vi "Add Subscriber.vi"(8 "error in (no error)":errorcluster, 10 "New FIFO Instance Config":T1, 11 "CIF_DAQ_DVR_Multi in":refnum<class "CIF_NIChn_DAQ.lvclass">) -> (0 "error out":errorcluster, 2 "New Publisher":string, 3 "CIF_DAQ_DVR_Multi out":refnum<class "CIF_NIChn_DAQ.lvclass">)   [LabVIEW 2021, in "CIF_NIChn_DAQ.lvclass"]
uses:
  CIF_NIChn_DAQ.lvclass
  CIF_NIChn_DAQ.lvclass/CIF_NIChn_DAQ.ctl
  CIFChannels/Typedef/Direction.ctl
  CIFChannels/CIFChannels.lvclass
  ChannelCommon/ChannelCommon.lvlib
  DAQ Base/CIF_NIChn_DAQ_Base.lvclass
  CIFChannels/Typedef/Channel State.ctl
  D:/dev/Packages/CIF_Channels_Core/src/CIF_NIChn/FIFO_DAQ/DAQ Base/CIF_NIChn_DAQ_Base.lvclass
  D:/dev/Packages/CIF_Channels_Core/src/CIF_NIChn/FIFO_U8/CIF_NIChn_Fifo_U8.lvclass
  D:/dev/Packages/CIF_Channels_Core/src/CIF_NIChn/NIChn/CIF_NIChn.lvclass
  D:/dev/Packages/CIF_Channels_Core/src/CIFChannels/CIFChannels.lvclass
  D:/dev/Packages/CIF_Channels_Core/src/CIF_NIChn/FIFO_DAQ/CIF_NIChn_DAQ.lvclass
  ChannelCommon/typedef/New FIFO Instance Configuration.ctl
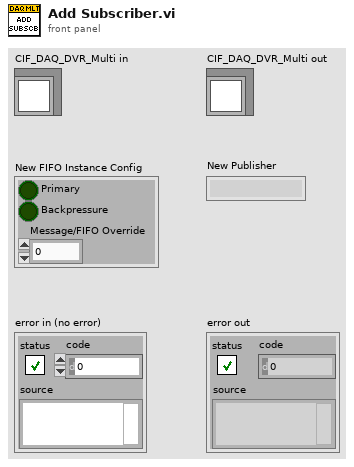
[diagram p1: front panel]
types:
  T1 = typedef "ChannelCommon.lvlib/New FIFO Instance Configuration.ctl" = cluster{"Primary":bool, "Backpressure":bool, "Message/FIFO Override":u32}
  T2 = typedef "CIFChannels.lvclass/Channel State.ctl" = enum16{"Creating", "Disconnected", "Connecting", "Connected", "Destroyed"}
  T3 = typedef "CIFChannels.lvclass/Direction.ctl" = enum16{"Publisher", "Subscriber"}
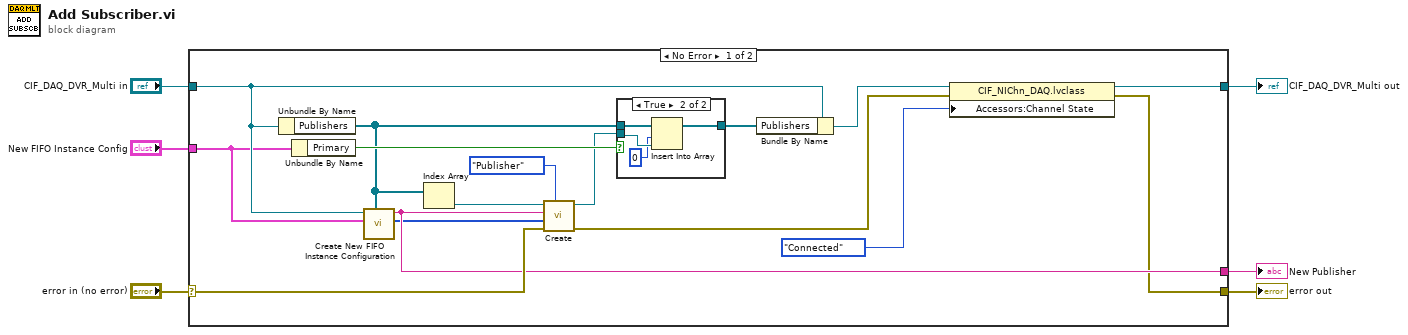
[diagram p0: block diagram]
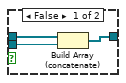
[diagram p2: hidden frame]
diagram:
  n1 = case shown="No Error" "error in (no error)" {
    selector: "error in (no error)" -> [w15 w31]
    tunnel: [w7 w31] -> w5
    tunnel: [w9 w30] -> w3
    tunnel: "CIF_DAQ_DVR_Multi in" -> [w17 w30]
    tunnel: "New FIFO Instance Config" -> [w16 _]
    tunnel: [w14 _] -> w1
    frame No Error {
      n2 = Unbundle By Name(w17) -> ("Publishers"=w12:refnum<class "CIF_NIChn_DAQ_Base.lvclass">[])
      n3 = Unbundle By Name(w16) -> ("Primary"=w20:bool)
      n4 = call "Create New FIFO Instance Configuration.vi"("Publisher Array in"=w12, "New FIFO Instance Config"=w16, "CIFChannels.lvclass"=w17) -> ("Flattened FIFO Config"=w13:u8[], "New Publisher"=w14:string)  [unwired: 7 in]
      n5 = Index Array(array=w12) -> (element=w22:refnum<class "CIF_NIChn_DAQ_Base.lvclass">)  [unwired: 1 in]
      n6 = call-dynamic "Create.vi"("Direction"=Direction."Publisher", "error in (no error)"=w15, "Custom Config Data"=w13, "Name"=w14, "CIF_NIChn_FIFO_DAQ in"=w22) -> ("error out"=w8:errorcluster, "CIF_NIChn_FIFO_DAQ out"=w18:refnum<class "CIF_NIChn_DAQ_Base.lvclass">)  [unwired: 5 in]
      n7 = case shown="True" w20 {
        tunnel: w12 -> [w25 w29]
        tunnel: [w24 w26] -> w19
        tunnel: w18 -> [w23 w28]
        frame False {
          n8 = Build Array (concatenate)(w25, w23) -> (w24:refnum<class "CIF_NIChn_DAQ_Base.lvclass">[])
        }
        frame True {
          n9 = Insert Into Array(array=w29, index=0, new element=w28) -> (w26:refnum<class "CIF_NIChn_DAQ_Base.lvclass">[])
        }
      }
      n10 = Bundle By Name(cluster=w17, "Publishers"=w19) -> (w10:refnum<class "CIF_NIChn_DAQ.lvclass">)
      n11 = property class="CIF_NIChn_DAQ.lvclass"(reference=w10, error in=w8, "Accessors:Channel State"=Channel_State."Connected" ("Channel State")) -> (reference out=w9:refnum<class "CIF_NIChn_DAQ.lvclass">, error out=w7:errorcluster)
    }
    frame Error {
    }
  }
  "error out" <- w5
  "CIF_DAQ_DVR_Multi out" <- w3
  "New Publisher" <- w1
